vi "kinetic simulation matrix-6.vi"() -> ()   [LabVIEW 2012]
uses:
  <vilib>/Utility/file.llb/Write To Spreadsheet File (DBL).vi
panel:
  in  "Fraction%":dbl=96.0 format="%#_2f"
  in  "kAF(um)2":dbl=0.22999999999999998 format="%#_6f"
  in  "k2 2":dbl=0.0005 format="%#_7f"
  in  "kF(um)2":dbl=0.064 format="%#_6f"
  in  "X2":dbl=0.0023000000000000004
  in  "one/two rates":bool=TRUE
  out "Efficency Summery Full":dbl[][](graph)=[[70.0, 85.77, 93.57, 97.4, 99.0], [79.3, 98.22, 97.643, 98.28, 98.22], [89.0, 95.66, 95.8, 96.0, 97.0], [90.0, 89.7, 90.6, 90.9, 90.5], [70.0, 85.77, 93.57, 97.4, 99.0], [79.3, 98.22, 97.643, 98.28, 98.22], [89.0, 95.66, 95.8, 96.0, 97.0], [90.0, 89.7, 90.6, 90.9, 90.5]]
  in  "Transition Matrix":i32[][](array[numeric])=[[1, 1, 2, 3, 3], [5, 2, 2, 3, 4], [0, 1, 3, 3, 4], [0, 0, 5, 4, 4], [1, 1, 2, 3, 3], [0, 1, 2, 2, 5], [0, 1, 1, 3, 4], [0, 0, 5, 4, 4]]
  in  "TP - S5":dbl[][](array[numeric])=[[999.0, 0.0, 0.0], [0.0, 0.0, 0.0], [0.0, 0.0, 0.0], [0.0, 0.0, 0.0], [999.0, 0.0, 0.0], [0.0, 0.0, 111.0], [0.0, 0.0, 0.0], [0.0, 0.0, 0.0]]
  in  "TP - S4":dbl[][](array[numeric])=[[0.0, 0.0, 0.0], [0.0, 0.0, 0.0], [0.0, 0.0, 0.0], [0.0, 111.0, 0.0], [0.0, 0.0, 0.0], [111.0, 0.0, 0.0], [0.0, 0.0, 0.0], [0.0, 111.0, 0.0]]
  in  "TP - S3":dbl[][](array[numeric])=[[0.0, 0.0, 0.0], [0.0, 0.0, 0.0], [0.0, 999.0, 0.0], [0.0, 0.0, 111.0], [0.0, 0.0, 0.0], [0.0, 0.0, 0.0], [999.0, 0.0, 0.0], [0.0, 0.0, 111.0]]
  in  "TP - S2":dbl[][](array[numeric])=[[0.0, 0.0, 0.0], [0.0, 111.0, 0.0], [0.0, 0.0, 0.0], [111.0, 0.0, 0.0], [0.0, 0.0, 0.0], [0.0, 0.0, 0.0], [0.0, 0.0, 0.0], [111.0, 0.0, 0.0]]
  in  "TP - S1":dbl[][](array[numeric])=[[0.0, 999.0, 0.0], [0.0, 0.0, 111.0], [0.0, 0.0, 0.0], [0.0, 0.0, 0.0], [0.0, 999.0, 0.0], [0.0, 0.0, 0.0], [0.0, 0.0, 0.0], [0.0, 0.0, 0.0]]
  in  "Start":bool
  in  "STOP All":bool
  out "kAF'":dbl=0.046
  in  "kAF(um)":dbl=0.22999999999999998 format="%#_6f"
  out "Simulated-Efficencys":dbl[][](array[numeric])=[[73.99155722326454, 98.68667917448406, 100.02345215759848, 100.02345215759848, 100.02345215759848], [97.37635705669481, 100.0301568154403, 100.0301568154403, 100.0301568154403, 100.0301568154403], [99.94562262098967, 100.05437737901033, 100.05437737901033, 100.05437737901033, 100.05437737901033], [100.07358351729212, 100.07358351729212, 100.07358351729212, 100.07358351729212, 100.07358351729212]]
  in  "State to Observe":i32=4
  in  "incubation time":dbl[](array[numeric])=[30.0, 100.0, 300.0, 1000.0, 3000.0] caption="Incubation time"
  in  "concentration (uM)":dbl[](array[numeric])=[0.2, 0.5, 1.0, 10.0]
  in  "Experamental-Efficencys":dbl[][](array[numeric])=[[70.95, 85.77, 93.57, 96.76, 98.88], [82.0, 94.6, 97.643, 98.28, 98.22], [89.0, 95.66, 95.8, 96.0, 97.0], [90.0, 89.7, 90.6, 91.9, 91.5]]
  out "Efficency Summery":dbl[][](graph)=[[70.0, 85.77, 93.57, 97.4, 99.0], [79.3, 98.22, 97.643, 98.28, 98.22], [89.0, 95.66, 95.8, 96.0, 97.0], [90.0, 89.7, 90.6, 90.9, 90.5], [25.493850167722698, 70.07614078057611, 97.26585378840318, 99.3251158085299, 99.3251158085299], [79.3, 98.22, 97.643, 98.28, 98.22], [89.0, 95.66, 95.8, 96.0, 97.0], [90.0, 89.7, 90.6, 90.9, 90.5]]
  in  "k2":dbl=0.135 format="%#_6f"
  out "AF/F":bool=TRUE
  in  "Matrix-Antifuel":dbl[][](array[numeric])=[[0.0, 0.0, 0.0, 0.0, 0.0, 0.0, 0.0, 0.0, 0.0, 0.0], [0.0, 0.0, 0.0, 0.0, 0.0, 0.0, 0.0, 0.0, 0.0, 0.0], [0.0, 0.0, 0.0, 0.0, 0.0, 0.0, 0.0, 0.0, 0.0, 0.0], [0.0, 0.0, 0.0, 0.0, 0.0, 0.0, 0.0, 0.0, 0.0, 0.0], [0.046, 0.0, 0.0, 0.0, 0.0, 0.0, 0.0, 0.0, 0.0, 0.0], [0.0, 0.0, 0.0, 0.0, 0.0, 0.0, 0.0, 0.0, 0.0, 0.0]]
  out "Concen (um)":dbl=0.2
  in  "kF(um)":dbl=0.064 format="%#_6f"
  out "kF'X":dbl=0.00048000000000000007
  in  "X":dbl=0.0024000000000000002
  out "kF'":dbl=0.0128
  out "nnew 2":i32=1
  out "inew 2":i32=1
  out "index_top 2":i32=2
  out "Final_A_index 2":i32[](array[numeric])=[0, 1, 2, 5, 2, 0, 0, 0, 0, 0]
  out "Final_D_index 2":i32[](array[numeric])=[0, 2, 1, 1, 4, 0, 0, 0, 0, 0]
  out "rate 2":dbl[](array[numeric])=[0.0, 0.0, 0.0, 0.0, 4000000000.000001, 0.0, 0.0, 0.0, 0.0, 0.0]
  in  "Matrix-Fuel":dbl[][](array[numeric])=[[0.0, 0.0, 0.0, 0.0, 0.0, 0.0, 0.0, 0.0, 0.0, 0.0], [0.0128, 0.0, 0.0, 0.0, 0.0, 0.0, 0.0, 0.0, 0.0, 0.0], [0.00048000000000000007, 0.0, 0.0, 0.0, 0.0, 0.0, 0.0, 0.0, 0.0, 0.0], [0.0, 0.00048000000000000007, 0.0128, 0.0, 0.0, 0.0, 0.0, 0.0, 0.0, 0.0], [0.0, 0.135, 0.135, 0.0, 0.0, 0.0, 0.0, 0.0, 0.0, 0.0], [0.0, 0.0, 0.0, 0.0, 0.0, 0.0, 0.0, 0.0, 0.0, 0.0]]
  in  "save?":bool
  out "nnew":i32=1
  out "inew":i32=1
  out "index_top":i32=2
  out "photime":dbl=9999.0
  out "srate":dbl
  out "time 2":dbl=0.30115000000000003
  out "Final_A_index":i32[](array[numeric])=[0, 1, 2, 5, 2, 0, 0, 0, 0, 0]
  out "Final_D_index":i32[](array[numeric])=[0, 2, 1, 1, 4, 0, 0, 0, 0, 0]
  out "rate":dbl[](array[numeric])=[0.0, 0.0, 0.0, 0.0, 333333000.0, 0.0, 0.0, 0.0, 0.0, 0.0]
  out "X-axes":dbl[](array[numeric])
  in  "time max":dbl=3000.0
  out "Kinetics":dbl[][](graph)
  in  "time per bin":dbl=0.1
  in  "NEXT":bool
  in  "number of state obs":i32=5
  out "Current pos":i32=5
  in  "start pos":i32
  out "probabilty distribution":dbl[](graph)=[5657697.888800734, 533641.3635606825, 18370.154266132402, 1479589.4928017345, 217688701.1005713, 0.0, 0.0, 0.0, 0.0, 0.0, 0.0, 0.0, 0.0]
  out "time":dbl=3000.0 format="%.3e"
  in  "stop inside":bool
  # "B"
  # "B"
  # "C'"
  # "D"
  # "C'"
  # "D"
  # "A"
  # "B'"
  # "A"
  # "B'"
  # "A"
  # "A"
  # "B"
  # "B"
  # "B'"
  # "B'"
  # "FUEL"
  # "C'"
  # "kF'"
  # "C'"
  # "D"
  # "ANTI-FUEL"
  # "D"
  # "kF'x"
  # "kF'"
  # "kF'x"
  # "k2"
  # "k2"
  # "200 nM"
  # "500 nM"
  # "1 uM"
  # "10 uM"
  # "30s"
  # "300s"
  # "3000s"
  # "100s"
  # "1000s"
  # "S1"
  # "S0"
  # "S2"
  # "S3"
  # "S4"
  # "999 - fuel efficency"
  # "111 antifuel efficency"
  # "F2"
  # "AF1"
  # "F3"
  # "AF2"
  # "F2"
  # "AF3"
  # "F1"
  # "AF2"
  # "right"
  # "lost"
  # "left"
  # "right"
  # "lost"
  # "left"
  # "right"
  # "lost"
  # "left"
  # "right"
  # "lost"
  # "right"
  # "lost"
  # "left"
  # "left"
  # "F2"
  # "F2"
  # "F2"
  # "F2"
  # "F2"
  # "AF1"
  # "AF1"
  # "AF1"
  # "AF1"
  # "AF1"
  # "F3"
  # "F3"
  # "F3"
  # "F3"
  # "F3"
  # "AF2"
  # "AF2"
  # "AF2"
  # "AF2"
  # "AF2"
  # "F2"
  # "F2"
  # "F2"
  # "F2"
  # "F2"
  # "AF3"
  # "AF3"
  # "AF3"
  # "AF3"
  # "AF3"
  # "F1"
  # "F1"
  # "F1"
  # "F1"
  # "F1"
  # "k1 B->D"
  # "AF2"
  # "AF2"
  # "AF2"
  # "AF2"
  # "AF2"
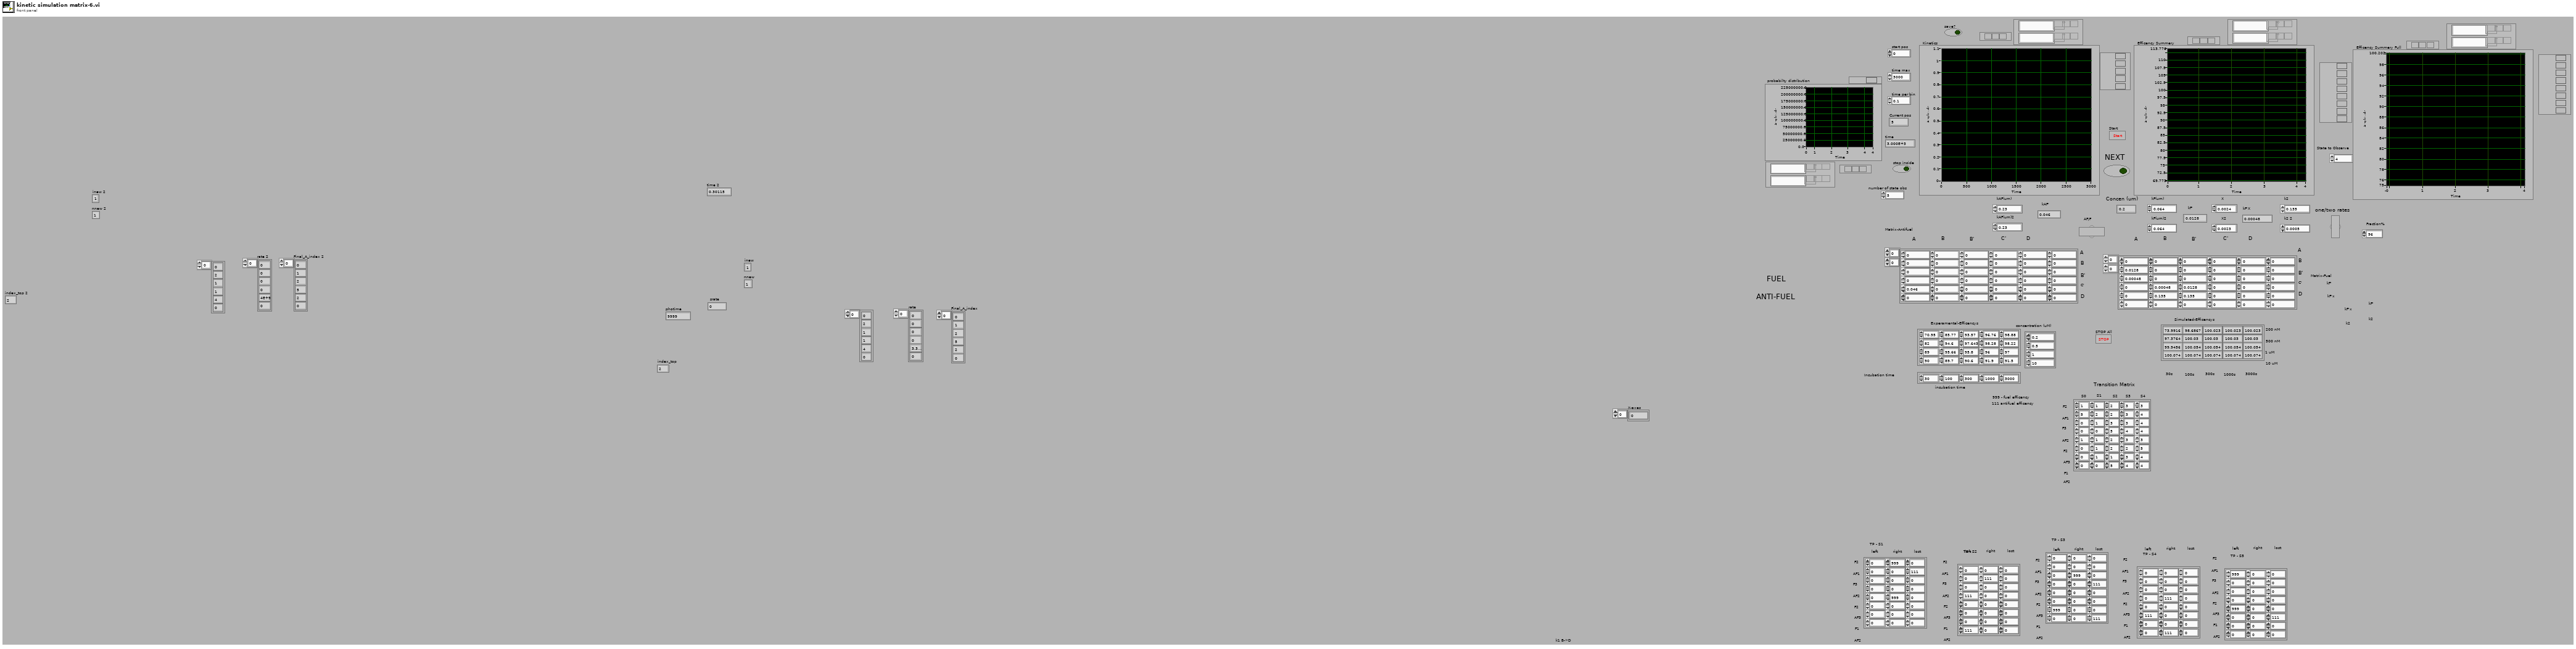
[diagram p1: front panel]
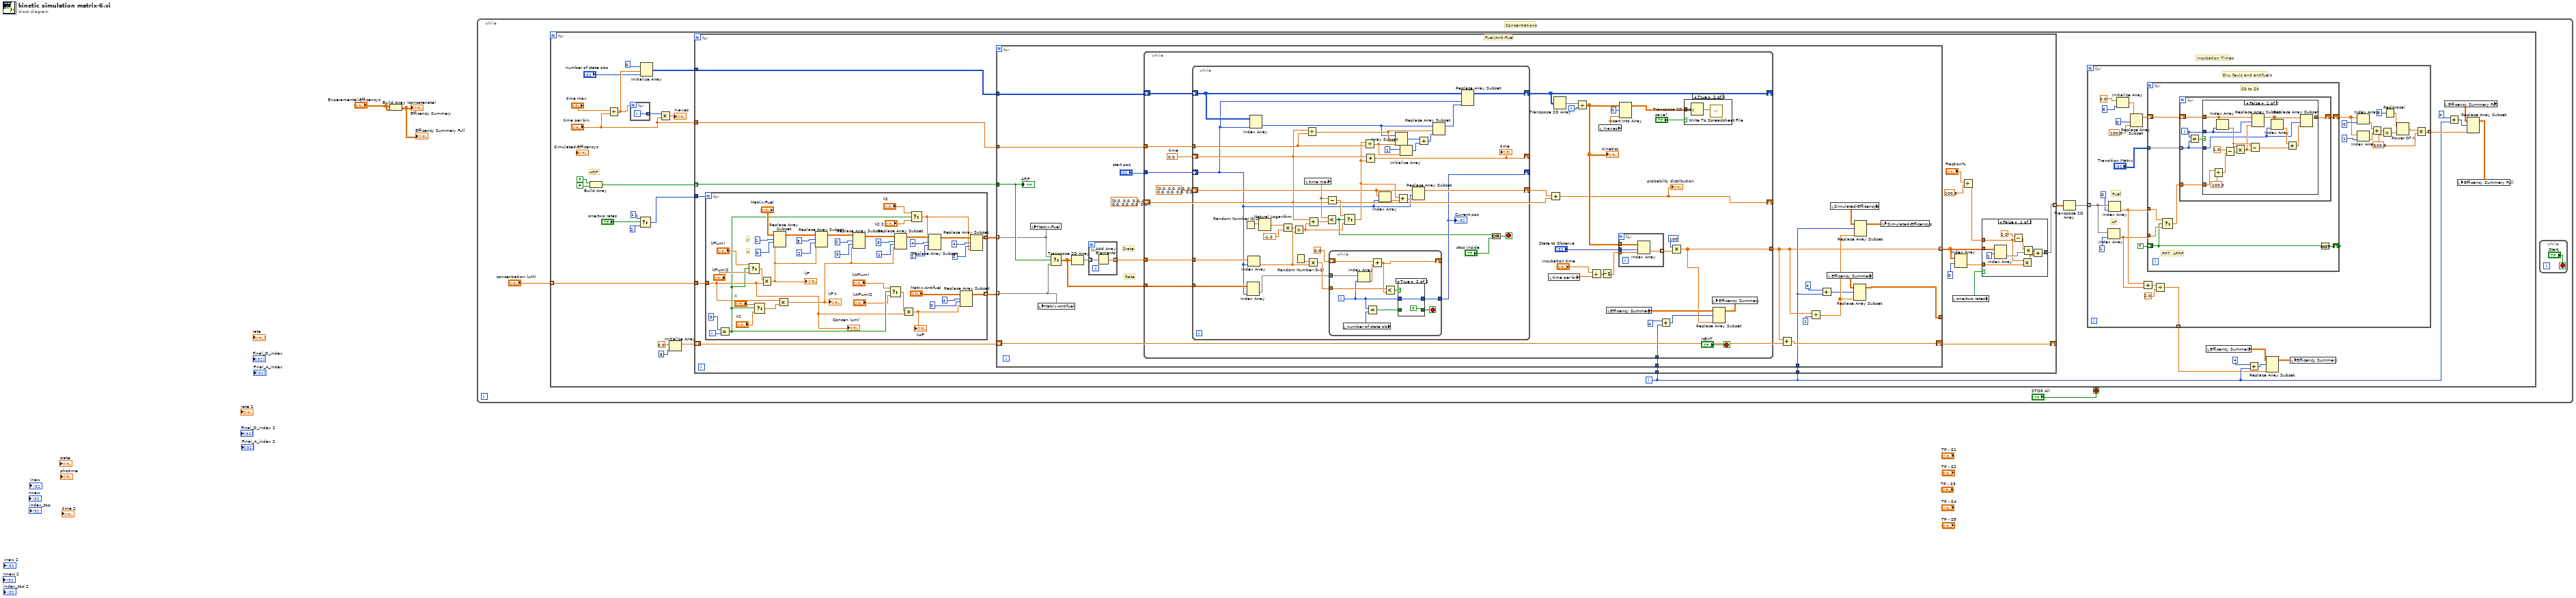
[diagram p0: block diagram]
diagram:
  n1 = Build Array (concatenate)("Experamental-Efficencys", "Experamental-Efficencys") -> (→"Efficency Summery" →"Efficency Summery Full":dbl[][])
  n2 = while {
    stop <- "STOP All" stop-if-true
    # "Concentrations"
    n3 = for {
      tunnel: "concentration (uM)" -> [w37] mode=indexing
      i -> [w7]
      # "AF/F"
      # "Incubation Times"
      n4 = Build Array(TRUE ("AF/F"), FALSE ("AF/F")) -> (w34:bool[])
      n5 = Divide(x="time max", y="time per bin") -> (x/y=w29:dbl)
      n6 = for {
        N: w29 -> [_]
        tunnel: [w284] -> w27 mode=indexing
        i -> [w284]
      }
      n7 = Select(t=1, s="one/two rates", f=2) -> (s? t:f=w17:i32)
      n8 = Initialize Array(0 ("dimension size"), w29, "number of state obs") -> (w19:i32[][])
      n9 = Multiply(x=w27, y="time per bin") -> (x*y=→"X-axes":dbl[])
      n10 = Initialize Array(0.0 ("element"), 5 ("dimension size")) -> (w25:dbl[])
      n11 = for {
        tunnel: w37 -> [w56]
        tunnel: w34 -> [w55] mode=indexing
        tunnel: w7 -> [w43]
        tunnel: [w44] -> w13 mode=indexing
        tunnel: w19 -> [w53]
        tunnel: "time per bin" -> [w52]
        shift-right: [w51] -> _
        shift-left: w25 -> [w54]
        tunnel: w17 -> [w48]
        tunnel: w7 -> [w47]
        # "Fuel/Anti-Fuel"
        n12 = for {
          N: w48 -> [_]
          tunnel: w56 -> [w68]
          tunnel: [w91] -> w50 mode=indexing
          tunnel: [w87] -> w49 mode=indexing
          i -> [w83]
          # "y"
          # "x"
          n13 = Equal?(x=0, y=w83) -> (x = y?=w69:bool)
          n14 = Select(t="kF(um)", s=w69, f="kF(um)2") -> (s? t:f=w79:dbl)
          n15 = Select(t="X", s=w69, f="X2") -> (s? t:f=w76:dbl)
          n16 = Multiply(x=w79, y=w68) -> (x*y=w85:dbl)
          "kF'" <- w85
          n17 = Replace Array Subset(array="Matrix-Fuel", new element=w85, index (row)=1, index (col)=0 ("disabled index (col)")) -> (w105:dbl[][])
          n18 = Multiply(x=w68, y=w76) -> (x*y=w86:dbl)
          "kF'X" <- w86
          n19 = Replace Array Subset(array=w105, new element=w85, index (row)=3, index (col)=2 ("disabled index (col)")) -> (w99:dbl[][])
          n20 = Replace Array Subset(array=w99, new element=w86, index (row)=2, index (col)=0 ("disabled index (col)")) -> (w100:dbl[][])
          n21 = Select(t="kAF(um)", s=w69, f="kAF(um)2") -> (s? t:f=w70:dbl)
          n22 = Replace Array Subset(array=w100, new element=w86, index (row)=3, index (col)=1 ("disabled index (col)")) -> (w93:dbl[][])
          n23 = Multiply(x=w70, y=w68) -> (x*y=w84:dbl)
          "kAF'" <- w84
          n24 = Select(t="k2", s=w69, f="k2 2") -> (s? t:f=w74:dbl)
          n25 = Replace Array Subset(array=w93, new element=w74, index (row)=4, index (col)=1 ("disabled index (col)")) -> (w94:dbl[][])
          n26 = Replace Array Subset(array="Matrix-Antifuel", new element=w84, index (row)=4, index (col)=0 ("disabled index (col)")) -> (w87:dbl[][])
          n27 = Replace Array Subset(array=w94, new element=w74, index (row)=4, index (col)=2 ("disabled index (col)")) -> (w91:dbl[][])
          "Concen (um)" <- w68
        }
        n28 = for {
          tunnel: w55 -> [w125]
          tunnel: w52 -> [w131]
          tunnel: w53 -> [w130]
          shift-right: [w118] -> w51
          shift-left: w54 -> [w124]
          tunnel: w47 -> [w113]
          tunnel: [w111] -> w46 mode=indexing
          tunnel: w50 -> [w115] mode=indexing
          tunnel: w49 -> [w114] mode=indexing
          tunnel: w43 -> [w112]
          tunnel: [w110] -> _
          # "Rate"
          # "Srate"
          n29 = local write "Matrix-Fuel"(w115) -> ()
          n30 = local write "Matrix-Antifuel"(w114) -> ()
          n31 = Select(t=w115, s=w125, f=w114) -> (s? t:f=w126:dbl[][])
          n32 = Transpose 2D Array(2D array=w126) -> (transposed array=w129:dbl[][])
          n33 = for {
            tunnel: w129 -> [w133] mode=indexing
            tunnel: [w134] -> w128 mode=indexing
            n34 = Add Array Elements(numeric array=w133) -> (sum=w134:dbl)
          }
          n35 = while {
            shift-right: [w136] -> _
            shift-left: dbl[] [0.0, 0.0, 0.0, 0.0, 0.0, 0.0, 0.0, 0.0, 0.0, 0.0, 0.0, 0.0, 0.0] ("Output Array") -> [w165]
            tunnel: w131 -> [w162]
            shift-right: [w159] -> _
            shift-left: w130 -> [w163]
            tunnel: w128 -> [w153]
            tunnel: w126 -> [w152]
            tunnel: "start pos" -> [w151]
            tunnel: [w137] -> w111
            tunnel: w112 -> [w135]
            i -> [w150]
            stop <- "NEXT" stop-if-true
            w161 = 0.0  # time
            n36 = while {
              shift-left: dbl[] [0.0, 0.0, 0.0, 0.0, 0.0, 0.0, 0.0, 0.0, 0.0, 0.0, 0.0, 0.0, 0.0] ("Output Array") -> [w205]
              shift-right: [w186] -> w158
              shift-left: w161 -> [w189]
              shift-right: [w184] -> _
              shift-left: w151 -> [w179]
              shift-right: [w175] -> _
              tunnel: w162 -> [w200]
              shift-right: [w187] -> w159
              shift-left: w163 -> [w193]
              tunnel: w153 -> [w181]
              tunnel: w152 -> [w180]
              stop <- w173 stop-if-true
              n37 = Random Number (0-1)() -> (number: 0 to 1=w210:dbl)
              n38 = Index Array(array=w180, index (col)=w179) -> (element=w176:dbl[])  [unwired: 1 in]
              n39 = Index Array(array=w181, index=w179) -> (element=w182:dbl)
              n40 = Index Array(array=w193, index (col)=w179) -> (element=w194:i32[])  [unwired: 1 in]
              n41 = Natural Logarithm(1:w210) -> (0:w209:dbl)
              n42 = Multiply(x=w209, y=-1.0) -> (x*y=w207:dbl)
              n43 = Divide(x=w207, y=w182) -> (x/y=w183:dbl)
              n44 = Random Number (0-1)() -> (number: 0 to 1=w206:dbl)
              n45 = local read "time max"() -> (w190:dbl)
              n46 = Divide(x=w189, y=w200) -> (x/y=w196:dbl)
              n47 = Multiply(x=w206, y=w182) -> (x*y=w177:dbl)
              n48 = Add(x=w189, y=w183) -> (x+y=w191:dbl)
              n49 = Less?(x=w190, y=w191) -> (x < y?=w174:bool)
              n50 = Subtract(x=w190, y=w189) -> (x-y=w188:dbl)
              n51 = while {
                shift-right: [w217] -> _
                shift-left: 0.0 -> [w220]
                tunnel: w177 -> [w218]
                tunnel: w176 -> [w214]
                tunnel: [w211] -> w175
                i -> [w213]
                stop <- w215 stop-if-true
                n52 = local read "number of state obs"() -> (w212:i32)
                n53 = Index Array(array=w214, index=w213) -> (element=w221:dbl)
                n54 = Equal?(x=w213, y=w212) -> (x = y?=w216:bool)
                n55 = Add(x=w220, y=w221) -> (x+y=w217:dbl)
                n56 = Less?(x=w218, y=w217) -> (x < y?=w219:bool)
                n57 = case shown="True" w219 {
                  tunnel: w213 -> [w222 w224]
                  tunnel: w216 -> [w223 _]
                  tunnel: [w223 TRUE] -> w215
                  tunnel: [w222 w224] -> w211
                  frame False {
                  }
                  frame True {
                  }
                }
              }
              "Current pos" <- w175
              n58 = Select(t=w188, s=w174, f=w183) -> (s? t:f=w185:dbl)
              n59 = Divide(x=w185, y=w200) -> (x/y=w195:dbl)
              n60 = Add(x=w189, y=w185) -> (x+y=w184:dbl)
              "time" <- w184
              n61 = Index Array(array=w205, index=w179) -> (element=w203:dbl)
              n62 = Array Subset(array=w194, index=w196, length=w195) -> (w199:i32[])
              n63 = Add(x=w185, y=w203) -> (x+y=w204:dbl)
              n64 = Initialize Array(1 ("dimension size"), w195) -> (w198:i32[])
              n65 = Replace Array Subset(array=w205, new element=w204, index=w179) -> (w186:dbl[])
              n66 = Add(x=w199, y=w198) -> (x+y=w197:i32[])
              n67 = Replace Array Subset(array=w194, new element=w197, index=w196) -> (w192:i32[])
              n68 = Replace Array Subset(array=w193, new element=w192, index (col)=w179) -> (w187:i32[][])  [unwired: 1 in]
              n69 = Or(x=w174, y="stop inside") -> (x .or. y?=w173:bool)
            }
            n70 = local read "time per bin"() -> (w146:dbl)
            n71 = Add(x=w158, y=w165) -> (x+y=w136:dbl[])
            "probabilty distribution" <- w136
            n72 = Transpose 2D Array(2D array=w159) -> (transposed array=w160:i32[][])
            n73 = Divide(x=w160, y=w150) -> (x/y=w147:dbl[][])
            "Kinetics" <- w147
            n74 = Divide(x="incubation time", y=w146) -> (x/y=w145:dbl[])
            n75 = local read "X-axes"() -> (w154:dbl[])
            n76 = Decrement(x=w145) -> (x-1=w143:dbl[])
            n77 = local read "Efficency Summery"() -> (w149:dbl[][])
            n78 = for {
              tunnel: w143 -> [w170] mode=indexing
              tunnel: [w169] -> w142 mode=indexing
              tunnel: "State to Observe" -> [w168]
              tunnel: w147 -> [w167]
              n79 = Index Array(array=w167, index (row)=w168, index (col)=w170) -> (element=w169:dbl)
            }
            n80 = Insert Into Array(array=w147, index (row)=0, new element=w154) -> (w156:dbl[][])  [unwired: 1 in]
            n81 = Add(x=4 ("index (row)"), y=w135) -> (x+y=w139:i32)
            n82 = Multiply(x=100 ("index (row)"), y=w142) -> (x*y=w137:dbl[])
            n83 = case shown="True" "save?" {
              tunnel: w156 -> [_ w172]
              frame False {
              }
              frame True {
                n84 = Transpose 2D Array(2D array=w172) -> (transposed array=w171:dbl[][])
                n85 = call-poly <vilib>:"Write To Spreadsheet File.vi"("2D data"=w171) -> ()  [unwired: 7 in, 1 out]
              }
            }
            n86 = Replace Array Subset(array=w149, new element=w137, index (row)=w139) -> (w141:dbl[][])  [unwired: 1 in]
            n87 = local write "Efficency Summery"(w141) -> ()
          }
          n88 = Add(x=w111, y=w124) -> (x+y=w118:dbl[])
          n89 = Divide(x=w111, y=1 ("index (row)")) -> (x/y=w117:dbl[])
          n90 = Add(x=4 ("index (row)"), y=w113) -> (x+y=w116:i32)
          n91 = local read "Efficency Summery"() -> (w122:dbl[][])
          n92 = local read "Simulated-Efficencys"() -> (w120:dbl[][])
          n93 = Replace Array Subset(array=w122, new element=w117, index (row)=w116) -> (w110:dbl[][])  [unwired: 1 in]
          n94 = Replace Array Subset(array=w120, new element=w117, index (row)=w113) -> (w121:dbl[][])  [unwired: 1 in]
          n95 = local write "Simulated-Efficencys"(w121) -> ()
          "AF/F" <- w125
        }
        n96 = local read "one/two rates"() -> (w39:bool)
        n97 = Index Array(array=w46, index (row)=0 ("y")) -> (element=w38:dbl[])  [unwired: 1 in]
        n98 = Divide(x="Fraction%", y=100.0) -> (x/y=w40:dbl)
        n99 = case shown="False" w39 {
          tunnel: w46 -> [w66 _]
          tunnel: [w60 w67] -> w44
          tunnel: w40 -> [w57 _]
          tunnel: w38 -> [w58 w67]
          frame False {
            n100 = Index Array(array=w66, index (row)=1 ("y")) -> (element=w64:dbl[])  [unwired: 1 in]
            n101 = Subtract(x=1.0 ("element"), y=w57) -> (x-y=w63:dbl)
            n102 = Multiply(x=w57, y=w58) -> (x*y=w59:dbl[])
            n103 = Multiply(x=w63, y=w64) -> (x*y=w61:dbl[])
            n104 = Add(x=w61, y=w59) -> (x+y=w60:dbl[])
          }
          frame True {
          }
        }
      }
      n105 = Transpose 2D Array(2D array=w13) -> (transposed array=w12:dbl[][])
      n106 = for {
        tunnel: w12 -> [w245] mode=indexing
        tunnel: [w231] -> w21 mode=indexing
        tunnel: [w226] -> w6 mode=indexing
        w232 = 100.0 ("element")
        # "thru feuls and antifuels"
        # "AF"
        # "Fuel"
        n107 = Index Array(array=w245, index=1 ("disabled index (col)")) -> (element=w229:dbl)
        n108 = Index Array(array=w245, index=0 ("disabled index (col)")) -> (element=w230:dbl)
        n109 = Initialize Array(0.0 ("element"), 6 ("dimension size")) -> (w251:dbl[])
        n110 = Replace Array Subset(array=w251, new element=100.0 ("element"), index=0) -> (w248:dbl[])
        n111 = Add(x=w230, y=w229) -> (x+y=w228:dbl)
        n112 = for {
          shift-right: [w255] -> w236
          shift-left: w248 -> [w256]
          tunnel: "Transition Matrix" -> [w261] mode=indexing
          tunnel: w230 -> [w259]
          tunnel: w229 -> [w258]
          shift-right: [w260] -> _
          shift-left: TRUE ("s") -> [w254]
          # "S0 to S4"
          # "F=T, AF=F"
          n113 = Select(t=w259, s=w254, f=w258) -> (s? t:f=w257:dbl)
          n114 = for {
            tunnel: w261 -> [w263] mode=indexing
            tunnel: w257 -> [w266]
            shift-right: [w262] -> w255
            shift-left: w256 -> [w265]
            i -> [w264]
            n115 = Equal?(x=w264, y=w263) -> (x = y?=w267:bool)
            n116 = case shown="False" w267 {
              tunnel: w266 -> [w282 _]
              tunnel: w265 -> [w280 w283]
              tunnel: w264 -> [w279 _]
              tunnel: w263 -> [w271 _]
              tunnel: [w269 w283] -> w262
              frame False {
                n117 = Divide(x=w282, y=100.0 ("element")) -> (x/y=w278:dbl)
                n118 = Index Array(array=w280, index=w279) -> (element=w275:dbl)
                n119 = Subtract(x=1.0, y=w278) -> (x-y=w276:dbl)
                n120 = Multiply(x=w275, y=w276) -> (x*y=w274:dbl)
                n121 = Subtract(x=w275, y=w274) -> (x-y=w268:dbl)
                n122 = Replace Array Subset(array=w280, new element=w274, index=w279) -> (w270:dbl[])
                n123 = Index Array(array=w270, index=w271) -> (element=w273:dbl)
                n124 = Add(x=w273, y=w268) -> (x+y=w272:dbl)
                n125 = Replace Array Subset(array=w270, new element=w272, index=w271) -> (w269:dbl[])
              }
              frame True {
                # "Stay at the same state"
              }
            }
          }
          n126 = Not(x=w254) -> (.not. x?=w260:bool)
        }
        n127 = Divide(x=w228, y=2.0) -> (x/y=w226:dbl)
        n128 = Index Array(array=w236, index=0 ("index (row)")) -> (element=w238:dbl)
        n129 = Index Array(array=w236, index=1 ("index (row)")) -> (element=w237:dbl)
        n130 = Add(x=w238, y=w237) -> (x+y=w235:dbl)
        n131 = Divide(x=w235, y=w232) -> (x/y=w234:dbl)
        n132 = Reciprocal(x=8 ("index (row)")) -> (1/x=w242:dbl)
        n133 = Power Of X(1:w234, 2:w242) -> (0:w233:dbl)
        n134 = Multiply(x=w233, y=w232) -> (x*y=w231:dbl)
      }
      n135 = local read "Efficency Summery"() -> (w8:dbl[][])
      n136 = Add(x=4 ("index (row)"), y=w7) -> (x+y=w10:i32)
      n137 = Replace Array Subset(array=w8, new element=w6, index (row)=w10) -> (w9:dbl[][])  [unwired: 1 in]
      n138 = local write "Efficency Summery"(w9) -> ()
      n139 = local read "Efficency Summery Full"() -> (w24:dbl[][])
      n140 = Add(x=4 ("index (row)"), y=w7) -> (x+y=w22:i32)
      n141 = Replace Array Subset(array=w24, new element=w21, index (row)=w22) -> (w20:dbl[][])  [unwired: 1 in]
      n142 = local write "Efficency Summery Full"(w20) -> ()
    }
    n143 = while {
      stop <- "Start" stop-if-true
    }
  }
